vi "close.vi"(8 "error in":errorcluster, 11 "TEC runtime in":refnum<class "TEC runtime.lvclass">) -> (0 "error out":errorcluster)   [LabVIEW 2013, in "TEC runtime.lvclass"]
doc: "Provides an interface for terminating a module instance. While this interface performs no operations, a child should close and deallocate any open references or memory."
uses:
  TEC runtime.lvclass
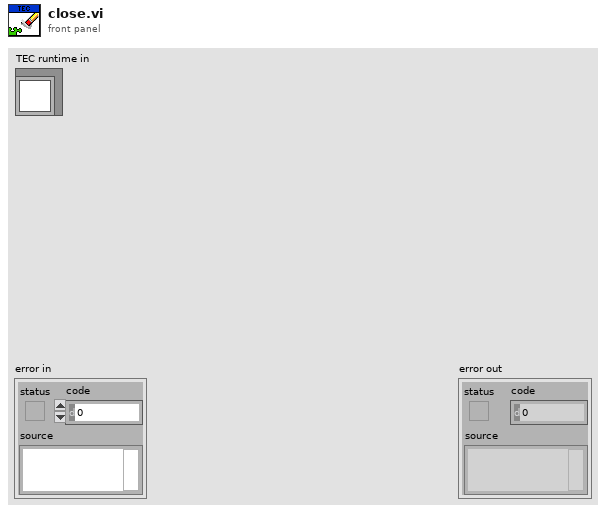
[diagram p1: front panel]
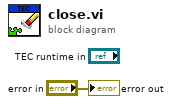
[diagram p0: block diagram]
diagram:
  "error out" <- "error in"
